vi "dialog_wait_close.vi"(0 "error in":errorcluster, 2 "milliseconds to wait":u32, 3 "async vi ref":refnum<vi>) -> ()   [LabVIEW 2020, in "varilib.lvlib"]
doc: "Closes assynchronously called wait dialog. Ignores error input. The 'milliseconds to wait' input delays closing of the dialog."
uses:
  varilib.lvlib
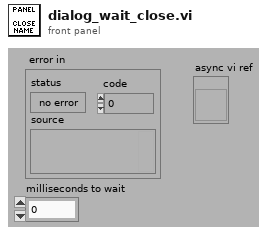
[diagram p1: front panel]
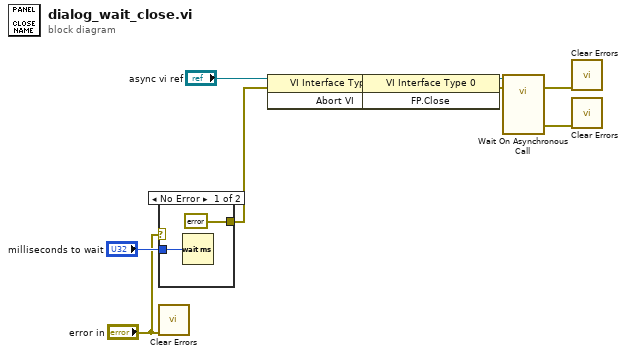
[diagram p0: block diagram]
diagram:
  n1 = case shown="No Error" "error in" {
    tunnel: "milliseconds to wait" -> [w12 _]
    tunnel: [errorcluster {"status"=FALSE, "code"=0, "source"=""} ("error in (no error)") _] -> w1
    frame No Error {
      n2 = Wait (ms)(milliseconds to wait=w12) -> ()  [unwired: 1 out]
    }
    frame Error {
    }
  }
  n3 = call <vilib>:"Clear Errors.vi"("error in (no error)"="error in") -> ()  [unwired: 5 in, 2 out]
  n4 = invoke class="VI Interface Type 0" method="Abort VI"(reference="async vi ref", error in=w1) -> (reference out=w4:refnum<vi>, error out=w5:errorcluster)  [unwired: 1 in, 1 out]
  n5 = invoke class="VI Interface Type 0" method="FP.Close"(reference=w4, error in=w5) -> (reference out=w8:refnum<vi>, error out=w9:errorcluster)  [unwired: 1 in, 1 out]
  n6 = call-by-ref "Wait On Asynchronous Call"(reference=w8, error in=w9) -> (error out=w7:errorcluster, 0:"error out"=w6:errorcluster)  [unwired: 11 in, 1 out]
  n7 = call <vilib>:"Clear Errors.vi"("error in (no error)"=w7) -> ()  [unwired: 5 in, 2 out]
  n8 = call <vilib>:"Clear Errors.vi"("error in (no error)"=w6) -> ()  [unwired: 5 in, 2 out]
